vi "OCV.vi"(0 "System no.":i32=1 min=1 max=4 step=1, 2 "Axes to move":string[](array[string]), 3 "Position values":dbl[](array[numeric]) format="%.6f", 5 "error in":errorcluster) -> (19 "error out":errorcluster)   [LabVIEW 2020]
doc: "OCV (Set Open-Loop Control Value)\n\nDescription\nSets control value directly to move the axis. Sensor feedback and control algorithms are not \ntaken into account.\nAll axes specified in the command start the motion simultaneously.\n\nFormat\nOCV{ <AxisID> <ControlValue>}\n\nArguments\n<AxisID>\nAn axis of the controller\nThe response to USG? CMD OCV indicates in the #Related Units block for which axes the \ncommand can be used.\nPossible values: Alias of the axis (p. 94) \n<ControlValue>\nControl value of the axis\nThe unit used for the control value is dependent on the type of axis.\nThe data format is float.\nPossible values: Dependent on the type of axis\n\nResponse\nnone\n\nExample\nAxis 1 is moved in open-loop operation by directly setting the control value with OCV. The axis \nis stopped with STP (p. 65) at the end of its travel range. Stopping sets the current control value \nto 0.\n>>eax?\n<<AXIS_1=0\n<<AXIS_2=0\n>>eax axis_1 1\n>>eax axis_2 1\n>>err?\n<<0 - (error 0 - \"No error\")\n>>eax?\n<<AXIS_1=1\n<<AXIS_2=1\n>>sam?\n<<AXIS_1=0x0\n<<AXIS_2=0x0\n>>ocv axis_1 1\n>>err?\n<<49156 - (error 49156 - \"User command level too low for\ncommand access\")\n>>ucl?\n<<USR\n>>ucl ADV advanced\n>>ucl?\n<<ADV\n>err?\n<<49169 - (error 49169 - \"Invalid mode of operation\")\n>>sam axis_1 0x1\n>>err?\n<<0 - (error 0 - \"No error\")\n>>ocv axis_1 1\n>>ocv?\n<<AXIS_1=1.0\n<<AXIS_2=0\n>>stp\n>>ocv?\n<<AXIS_1=0\n<<AXIS_2=0\n>>err?\n<<0 - (error 0 - \"No error\")\n>>sam? axis_1\n<<AXIS_1=0x1\n\nNotes\nMotion is only executed if the active user command level (p. 69) is at least ADV and if the \nfollowing conditions are fulfilled for all specified axes:\n- The axis is in the Operation enabled state.\n- An open-loop mode of operation ? 0x00 is set. For details on permitted modes of \noperation, see \"Motion Behavior - GCS 3.0\" (p. 101). \nFor further details, see \"Drive State Machine\" (p. 101) and the status register of the axis (p. 97). \nThe STV? command (p. 66) queries the status register.\nThe current control value can be queried with the commands OCV? (p. 29) or SPV? RAM Axis_n\n- 0x109 (p. 63). \nMotion can be stopped with the STP (p. 65) and HLT (p. 19) commands.\n\nLimitation of the control value: The controller does not check whether the control value is valid \nwhen it is entered with OCV. A check is only carried out when the control value specification is \nimplemented in the container unit \"Drive\". There, the specification is limited to the maximum \nor minimum permitted value. The axis moves using the limited control value and a \ncorresponding warning can be queried with LOG? (p. 21) (also displayed in the status register of \nthe system (p. 99), bit 3 \"Warning\"). The limitation is based on the following parameters of the \ncontainer unit \"Drive\", illustrated using drive 1 as an example:\n<<DRV_1 - 0x106 FLOAT32 - USR USR 30.0E-3 \n300.0E-3 Configuration Input Limit Max - - \n<<DRV_1 - 0x107 FLOAT32 - USR USR -300.0E3 -30.0E-3 Configuration Input Limit Min -\nFor further information, see \"Motion Behavior - GCS 3.0\" (p. 101). \n\nUser command level\nADV"
panel:
  # "OCV (Set Open-Loop Control Value)\n\nSets control value directly to move the axis. Sensor feedback and control algorithms are not  taken into account.\nAll axes specified in the command start the motion simultaneously."
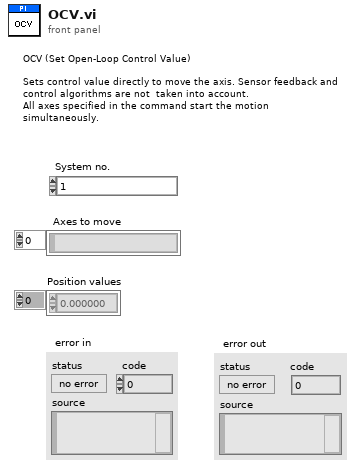
[diagram p1: front panel]
types:
  T1 = typedef "Syntax.ctl" = enum16{"GCS 1.0", "GCS 2.0", "GCS 3.0"}
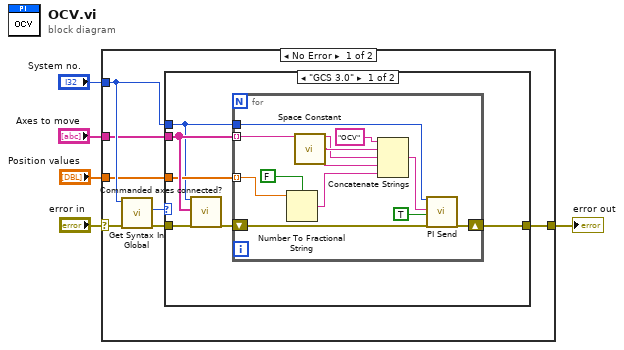
[diagram p0: block diagram]
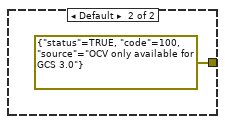
[diagram p2: hidden frame]
diagram:
  n1 = case shown="No Error" "error in" {
    selector: "error in" -> [w10 w31]
    tunnel: [w9 w31] -> w4
    tunnel: "Axes to move" -> [w7 _]
    tunnel: "System no." -> [w8 _]
    tunnel: "Position values" -> [w6 _]
    frame No Error {
      n2 = call "Get Syntax In Global.vi"("error in"=w10, "System no."=w8) -> ("error out"=w11:errorcluster, "Syntax"=w12:T1)  [unwired: 8 in]
      n3 = case shown="\"GCS 3.0\"" w12 {
        tunnel: [w14 errorcluster {"status"=TRUE, "code"=100, "source"="OCV only available for GCS 3.0"} ("error out")] -> w9
        tunnel: w11 -> [w17 _]
        tunnel: w8 -> [w13 _]
        tunnel: w7 -> [w16 _]
        tunnel: w6 -> [w15 _]
        frame "GCS 3.0" {
          n4 = call "Commanded axes connected?.vi"("System no."=w13, "Commanded axes"=w16, "error in"=w17) -> ("error out"=w18:errorcluster)  [unwired: 16 out]
          n5 = for {
            shift-right: [w29] -> w14
            shift-left: w18 -> [w28]
            tunnel: w16 -> [w23] mode=indexing
            tunnel: w15 -> [w20] mode=indexing
            tunnel: w13 -> [w19]
            n6 = Number To Fractional String(use system decimal point (T)=FALSE, number=w20) -> (F-format string=w21:string)  [unwired: 2 in]
            n7 = call <vilib>:"Space Constant.vi"() -> ("String"=w24:string)
            n8 = Concatenate Strings("OCV", w24, w23, w24, w21) -> (w25:string)
            n9 = call "PI Send.vi"("System no."=w19, "String to send"=w25, "Attach termination char.?"=TRUE ("Attach Linefeed?"), "error in"=w28) -> ("error out"=w29:errorcluster)  [unwired: 2 in, 13 out]
          }
        }
        frame Default {
        }
      }
    }
    frame Error {
    }
  }
  "error out" <- w4
